vi "AnalogicMeas.vi"() -> ()   [LabVIEW 2017]
uses:
  DefDeType/ListeMachineEtats.ctl
  <vilib>/DAQmx/read.llb/DAQmx Read (Analog 1D Wfm NChan NSamp).vi
  DefDeType/WhichPath.ctl
  <vilib>/DAQmx/write.llb/DAQmx Write (Digital Bool 1Line 1Point).vi
  DefDeType/ClusterRefCtrlUSBB.ctl
  <vilib>/DAQmx/create/channels.llb/DAQmx Create Channel (DO-Digital Output).vi
  <vilib>/DAQmx/configure/trigger.llb/DAQmx Start Trigger (Digital Edge).vi
  <vilib>/DAQmx/configure/task.llb/DAQmx Configure Logging (TDMS).vi
panel:
  in  "Reprocess":bool
  in  "Calibration":bool
  out "Graph2":waveform(dbl)[](graph)
  in  "NextTest Num":u32
  out "num iteration":i32
  out "Acquisition Time":dbl(slide) max=10.0 scale=0.0..1000.0
  in  "ModifConfig":bool
  out "Test List":i32(listbox)=-1
  in  "Bouton Stop":bool
  in  "Bouton Rec":bool
  out "Projet :":string
  out "message":string
  in  "Bouton Quit":bool
  out "LoopTime":u32(graph)
  out "Graph1":waveform(dbl)[](graph)
  # "Analogic Measurements"
  # "Project"
  # "Actions"
  # "Test List"
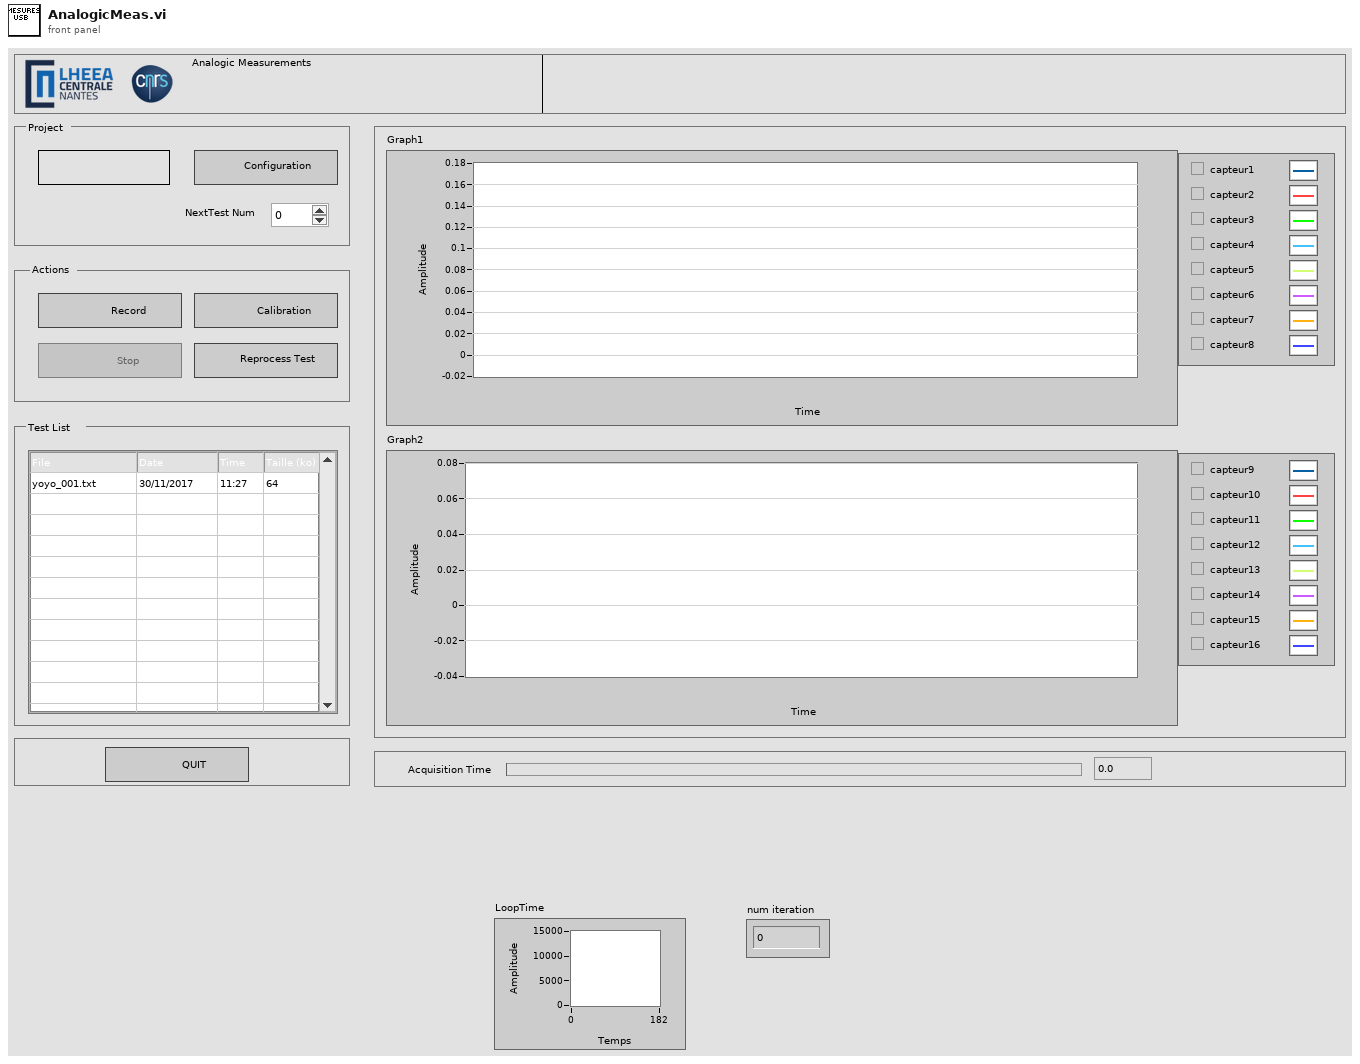
[diagram p1: front panel]
types:
  T1 = typedef "ClusterRefCtrlUSBB.ctl" = cluster{"Reprocess":refnum<vi>, "ModifConfig":refnum<vi>, "Bouton Rec":refnum<vi>, "Bouton Stop":refnum<vi>, "Bouton Quit":refnum<vi>, "Calibration":refnum<vi>, "Test List":refnum<vi>, "NextTest Num":refnum<vi>, "message":refnum<vi>}
  T2 = typedef "ListeMachineEtats.ctl" = enum16{"Init", "NewProj", "OpenProj", "InitLect", "Lect", "InitRec", "Rec", "Processing", "Quit"}
  T3 = cluster{"Graph2Index":i32[], "Graph1Index":i32[]}
  T4 = enum8{"Enabled", "Disabled", "Disabled and Grayed Out"}
  T5 = enum32{"Invalid", "Standard", "Closed", "Hidden", "Minimized", "Maximized"}
  T6 = typedef "WhichPath.ctl" = enum16{"DossierProjet", "Config", "Meas", "MeasPCI", "MeasCRIO1", "MeasCRIO2", "MeasQualisys", "MeasHBM", "MeasTDMS", "Fig", "Res"}
  T7 = typedef "WhichPath.ctl" = enum16{"DossierProjet", "Config", "Meas", "MeasSuitCase", "MeasOnBoard", "MeasQualisys", "MeasTDMS", "MeasHexapode", "MeasNortek", "Fig", "Res", "MeasUSB"}
  T8 = typedef "ConfigTotale.ctl" = cluster{"VoltageChannels":T9, "WheastoneBridgeChannels":T10, "Configuration":T11}
  T9 = typedef "VoltageChannels.ctl" = cluster{"ChannelNames":string[], "Sensitivity(Unit/V)":dbl[], "AutoZero":bool[], "ChannelUnits":string[], "Offsets(Units)":dbl[], "Graph Num":u8[]}
  T10 = typedef "WBridgeChannels.ctl" = cluster{"ChannelNames":string[], "Sensitivity(Unit/V)":dbl[], "AutoZero":bool[], "ChannelUnits":string[], "Offsets(Units)":dbl[], "Graph Num":u8[]}
  T11 = typedef "Configuration.ctl" = cluster{"AcqSamplingRate(Hz)":u32, "AcqTime(s)":u32, "Trigger":bool, "NbVoltageChannels":u32, "NbWBridgeChannels":u32, "Qualisys":bool, "Hexapode":bool, "FinalSamplingRate(Hz)":u32, "QualisysDataType":enum16{"6DOF", "3DTracking", "6DOF + 3D"}, "Nortek":bool, "HBM":bool}
  T12 = cluster{"Acquisition Time":refnum<vi>, "Graph1":refnum<vi>, "Graph2":refnum<vi>}
  T13 = typedef "MergeFileConfig.ctl" = cluster{"Test Num : ":u32, "Project :":string, "Qualisys file":path, "HBM file":path, "QualisysDataType":enum16{"6DOF", "3DTracking", "6DOF + 3D"}, "Qualisys":bool, "HBM":bool}
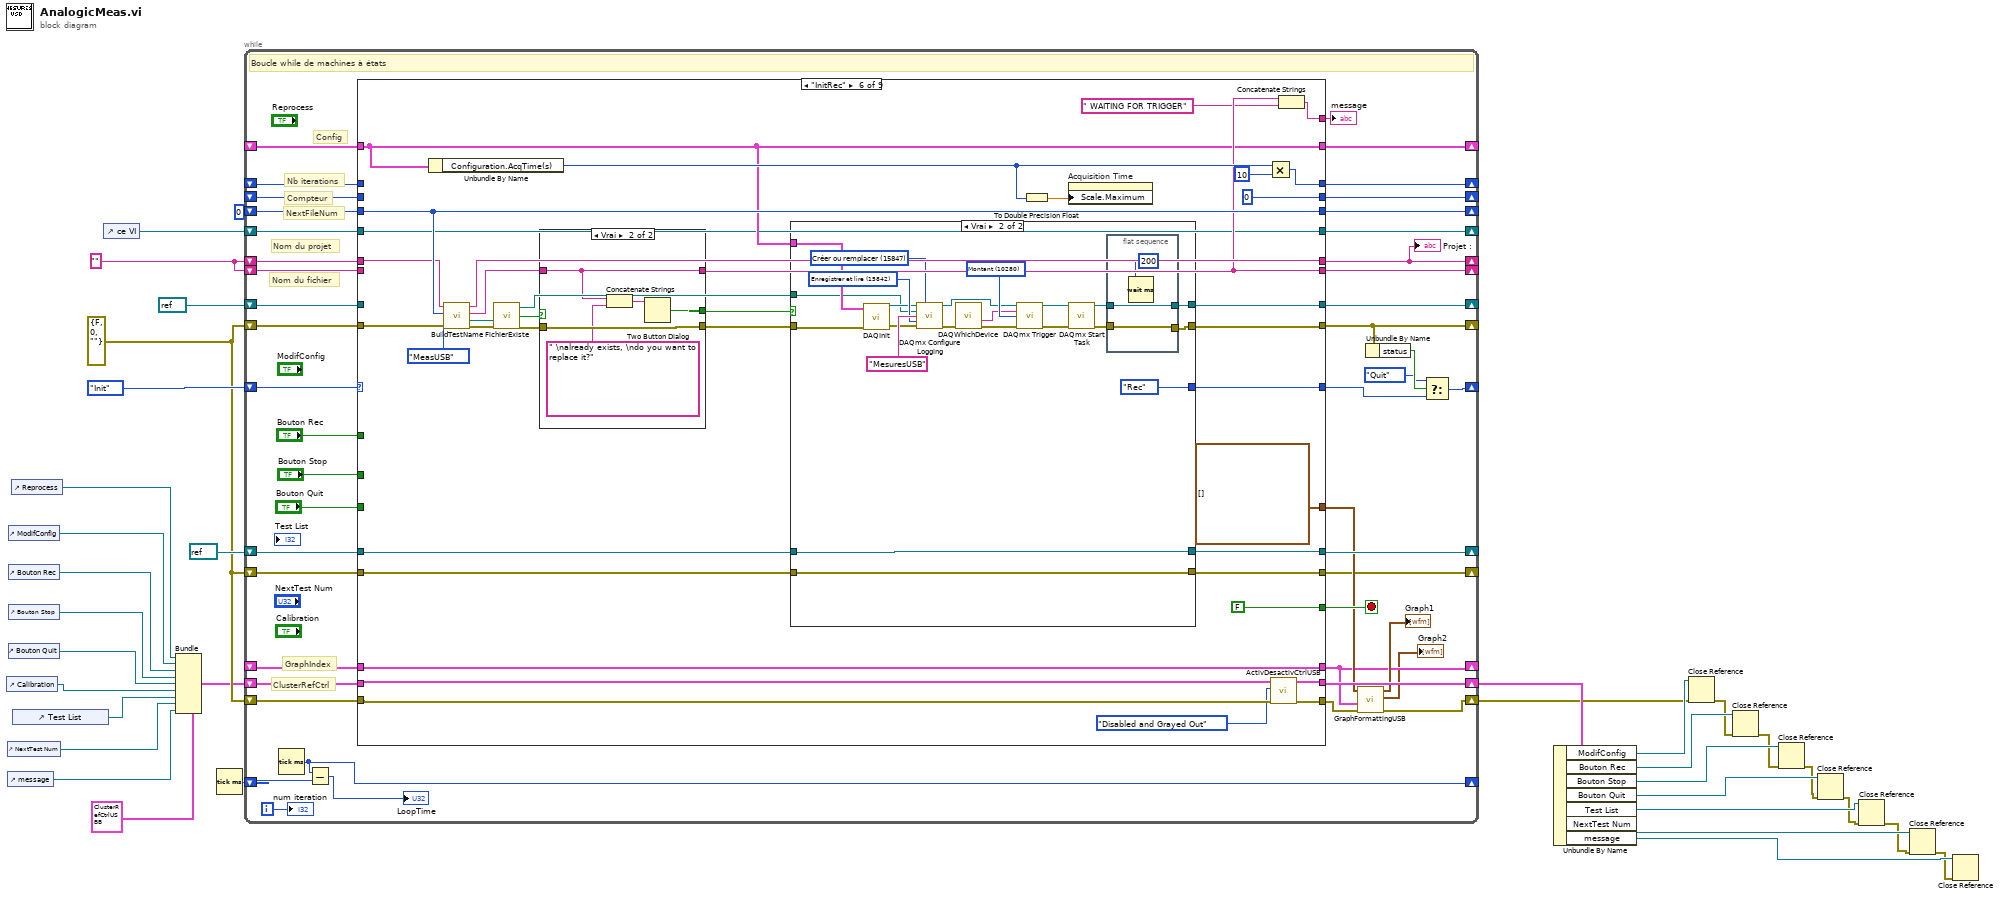
[diagram p0: block diagram]
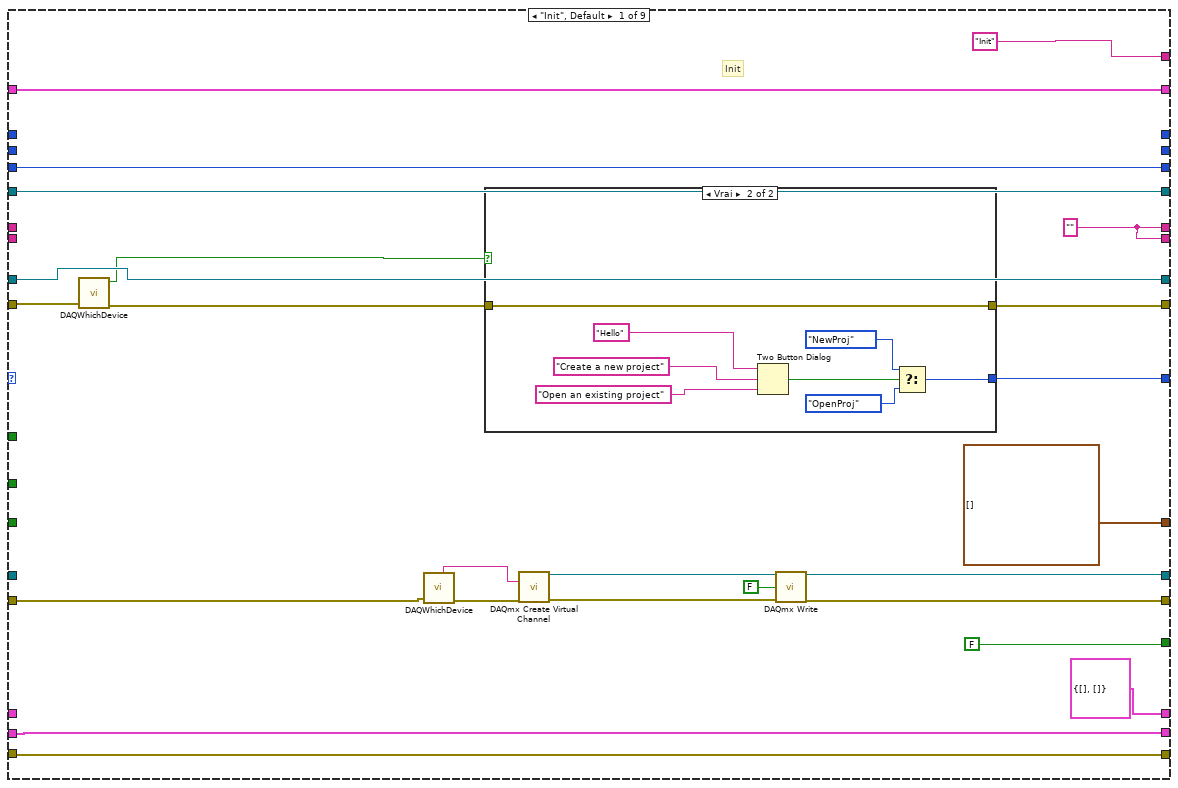
[diagram p2: hidden frame]
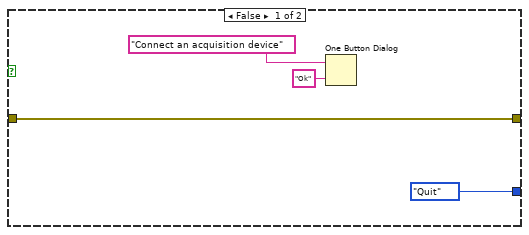
[diagram p3: hidden frame]
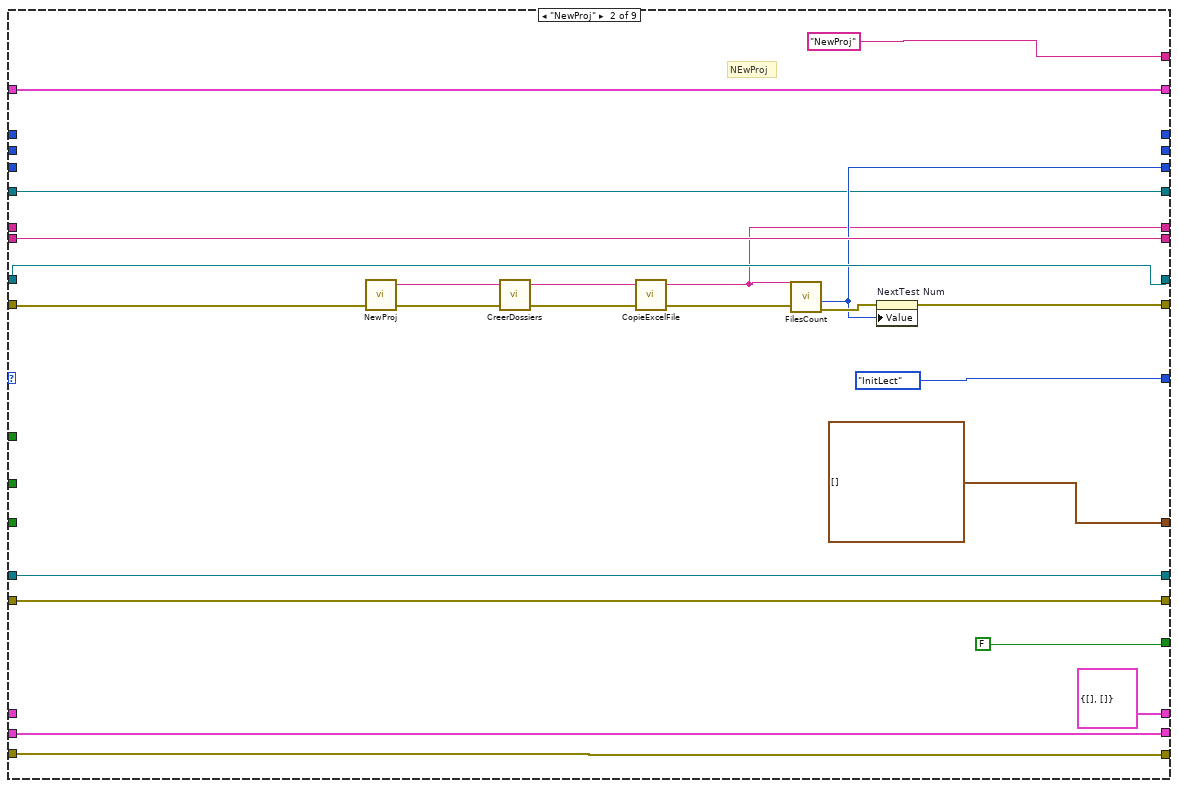
[diagram p4: hidden frame]
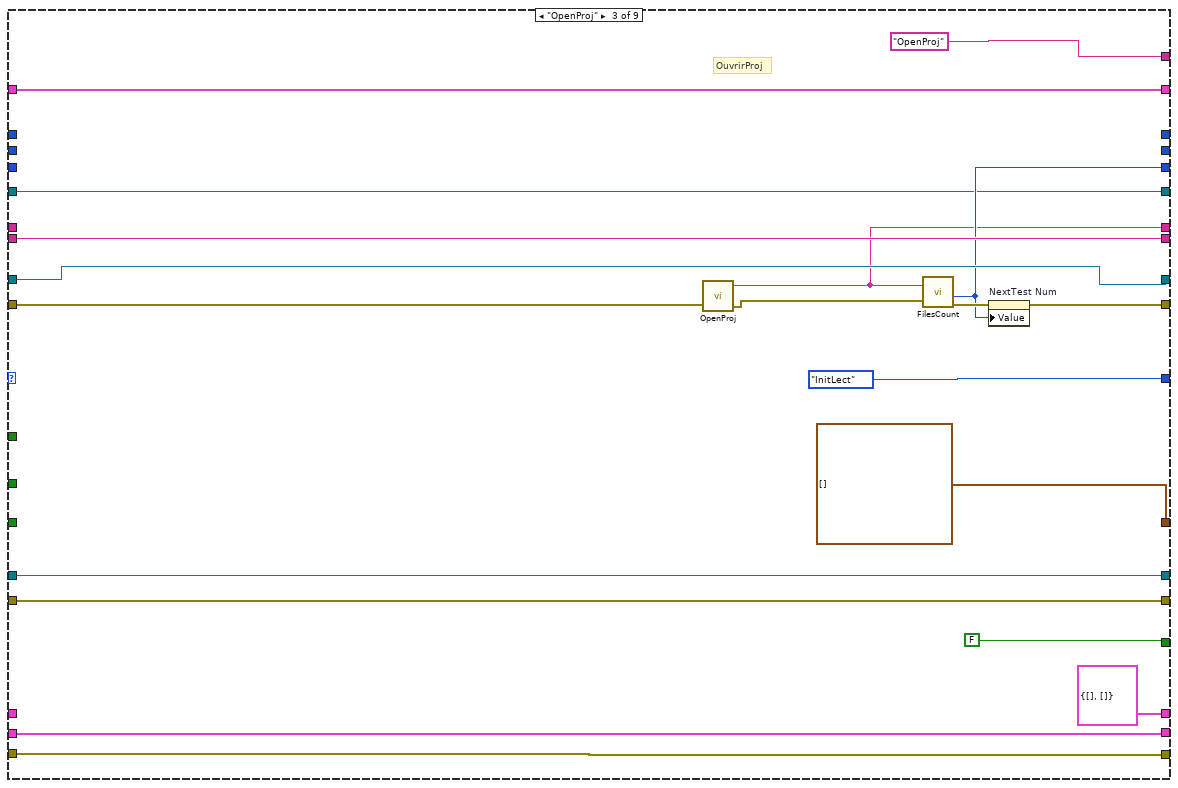
[diagram p5: hidden frame]
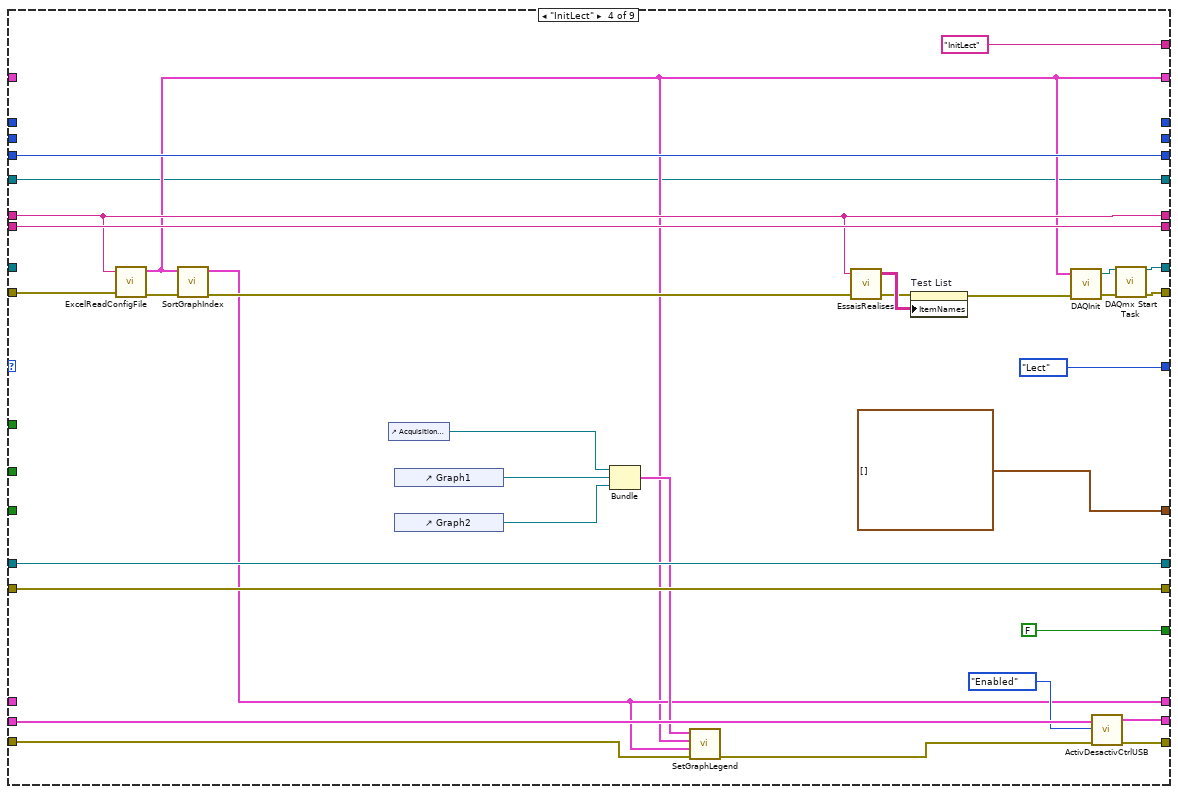
[diagram p6: hidden frame]
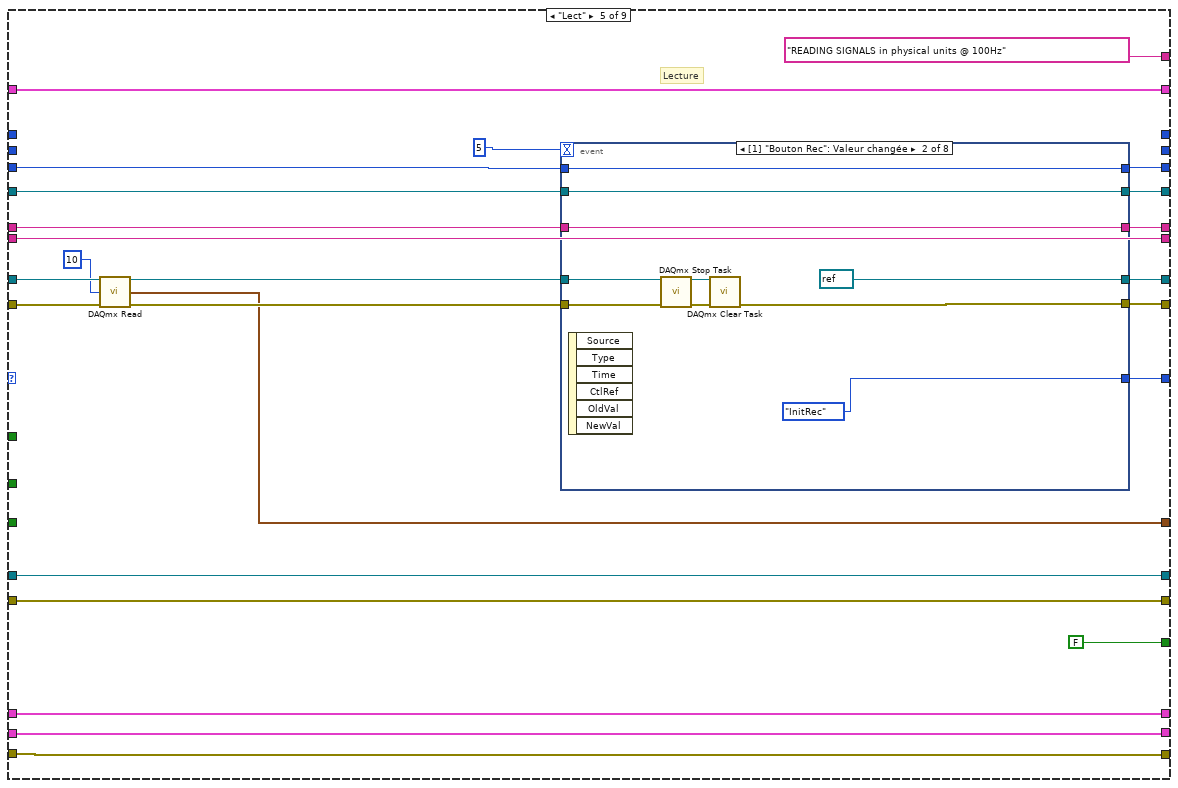
[diagram p7: hidden frame]
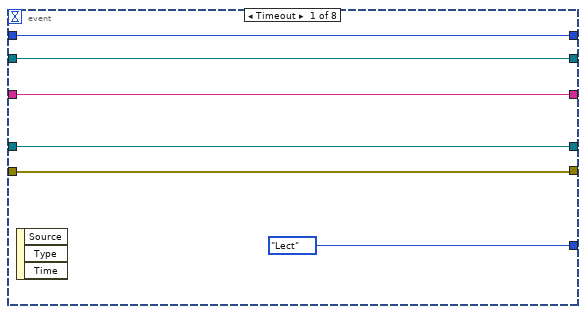
[diagram p8: hidden frame]
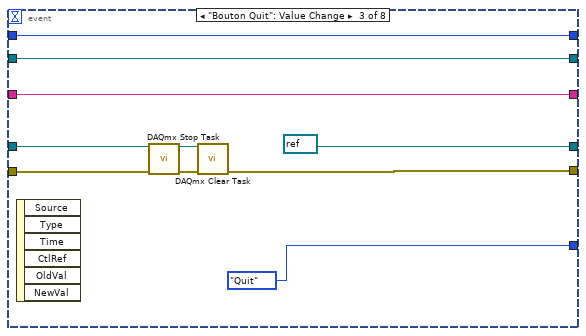
[diagram p9: hidden frame]
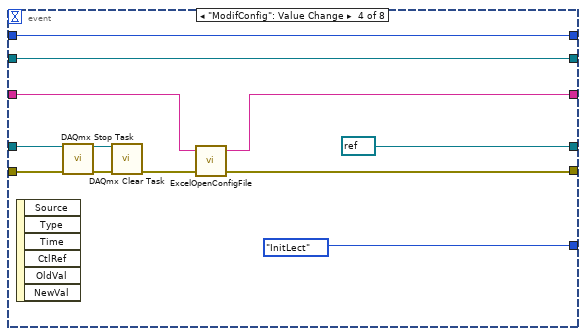
[diagram p10: hidden frame]
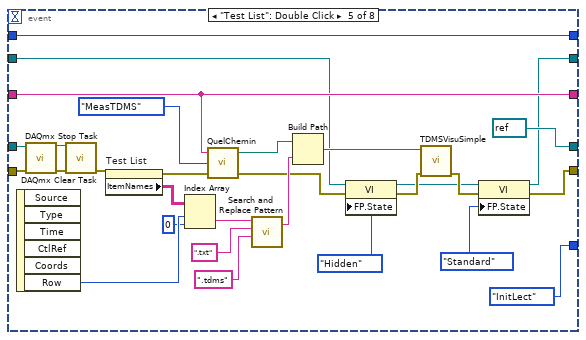
[diagram p11: hidden frame]
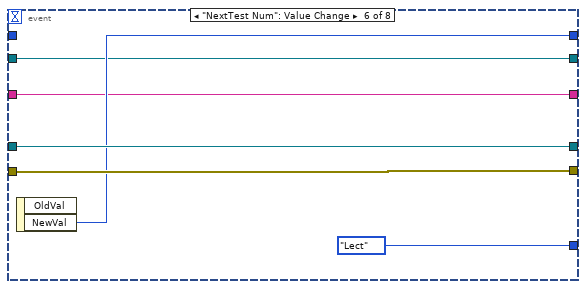
[diagram p12: hidden frame]
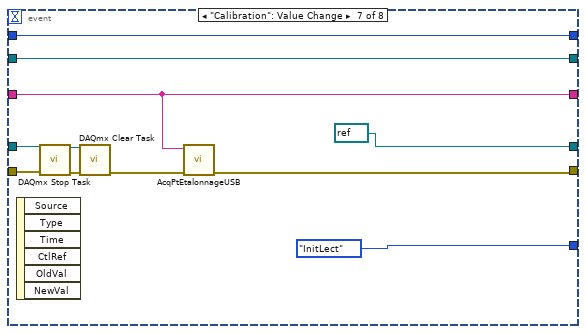
[diagram p13: hidden frame]
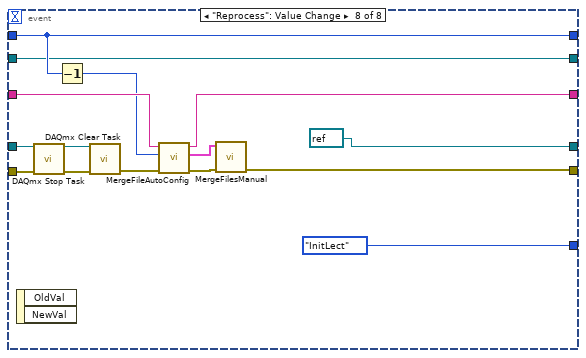
[diagram p14: hidden frame]
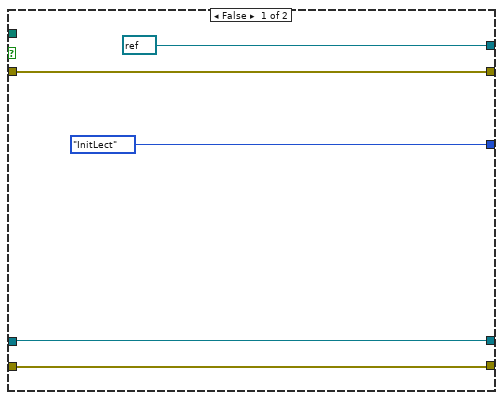
[diagram p15: hidden frame]
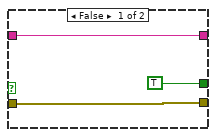
[diagram p16: hidden frame]
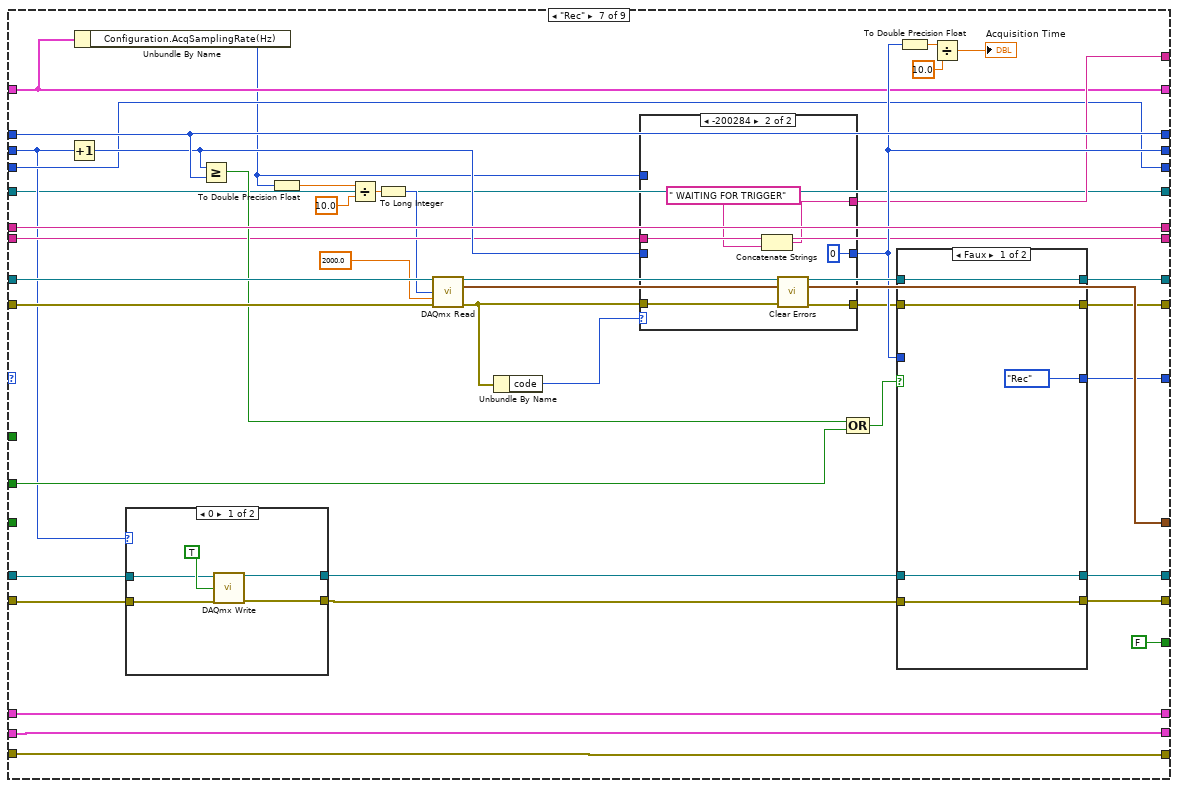
[diagram p17: hidden frame]
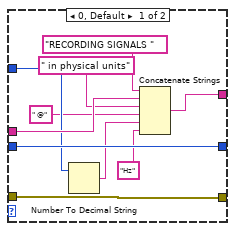
[diagram p19: hidden frame]
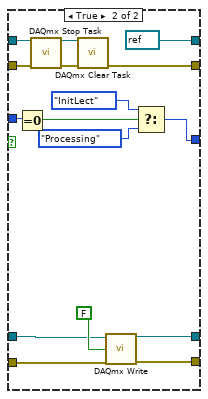
[diagram p20: hidden frame]
diagram:
  w29 = "" ("NomProjetOUT")
  w28 = errorcluster {"status"=FALSE, "code"=0, "source"=""} ("error out")
  n1 = control-ref of="Calibration"() -> (w5:refnum<vi>)
  n2 = control-ref of="NextTest Num"() -> (w22:refnum<vi>)
  n3 = control-ref of="message"() -> (w21:refnum<vi>)
  n4 = control-ref of="ModifConfig"() -> (w27:refnum<vi>)
  n5 = control-ref of="Bouton Rec"() -> (w26:refnum<vi>)
  n6 = control-ref of="Bouton Stop"() -> (w25:refnum<vi>)
  n7 = control-ref of="Bouton Quit"() -> (w24:refnum<vi>)
  n8 = control-ref of="Reprocess"() -> (w4:refnum<vi>)
  n9 = control-ref of="Test List"() -> (w23:refnum<vi>)
  n10 = control-ref of="ce VI"() -> (w1:refnum<vi>)
  n11 = Bundle(cluster=T1 {"Reprocess"=refnum, "ModifConfig"=refnum, "Bouton Rec"=refnum, "Bouton Stop"=refnum, "Bouton Quit"=refnum, "Calibration"=refnum, "Test List"=refnum, "NextTest Num"=refnum, "message"=refnum} ("ClusterRefCtrl"), "Reprocess"=w4, "ModifConfig"=w27, "Bouton Rec"=w26, "Bouton Stop"=w25, "Bouton Quit"=w24, "Calibration"=w5, "Test List"=w23, "NextTest Num"=w22, "message"=w21) -> (w2:T1)
  n12 = Tick Count (ms)() -> (millisecond timer value=w33:u32)
  n13 = while {
    shift-right: [w40] -> _
    shift-left: ListeMachineEtats."Init" ("ListeMachineEtats") -> [w61]
    shift-right: [w52] -> _
    shift-left: w29 -> [w79]
    shift-right: [w39] -> _
    shift-left: w28 -> [w78]
    shift-right: [w77] -> _
    shift-left: refnum<k21> refnum ("task out") -> [w76]
    shift-right: [w71] -> _
    shift-left: w29 -> [w70]
    shift-right: [w68] -> _
    shift-left: w33 -> [w69]
    shift-right: [w38] -> _
    shift-left: w28 -> [w66]
    shift-right: [w65] -> _
    shift-left: refnum<k21> refnum ("task out") -> [w64]
    shift-right: [w63] -> _
    shift-left: _ -> [w62]
    shift-right: [w37] -> w12
    shift-left: w28 -> [w60]
    shift-right: [w59] -> _
    shift-left: _ -> [w58]
    shift-right: [w57] -> _
    shift-left: _ -> [w56]
    shift-right: [w54] -> _
    shift-left: u32 0 ("NewVal") -> [w53]
    shift-right: [w50] -> w20
    shift-left: w2 -> [w51]
    shift-right: [w45] -> _
    shift-left: _ -> [w49]
    shift-right: [w35] -> _
    shift-left: w1 -> [w36]
    i -> [w55]
    stop <- w75 stop-if-true
    # "ClusterRefCtrl"
    # "GraphIndex"
    # "NextFileNum"
    # "Compteur"
    # "Nb iterations"
    # "Config"
    # "Nom du fichier"
    # "Nom du projet"
    # "Boucle while de machines à états"
    n14 = Tick Count (ms)() -> (millisecond timer value=w68:u32)
    n15 = Subtract(x=w68, y=w69) -> (x-y=→"LoopTime":u32)
    n16 = case shown="\"InitRec\"" w61 {
      tunnel: [w104 ListeMachineEtats."InitLect" ("ListeMachineEtats") ListeMachineEtats."InitLect" ("ListeMachineEtats") ListeMachineEtats."Lect" ("ListeMachineEtats") w205 w344 w425 ListeMachineEtats."InitLect" ("ListeMachineEtats") ListeMachineEtats."Init" ("ListeMachineEtats")] -> w42
      tunnel: ["Init" ("message") "NewProj" ("message") "OpenProj" ("message") "InitLect" ("message") "READING SIGNALS in physical units @ 100Hz" ("message") w343 w406 "Data Processing" ("message") "Quitter" ("message")] -> w80
      tunnel: [w93 w120 w143 w176 w198 w331 w424 w485 w528] -> w52
      tunnel: w79 -> [_ _ _ w176 w204 w332 w424 w489 _]
      tunnel: [w96 w123 w145 w183 w207 w349 w426 w494 w507] -> w39
      tunnel: w78 -> [w99 w134 w157 w177 w213 w335 w432 w490 w513]
      tunnel: [w102 w133 w156 w185 w206 w350 w427 refnum<k21> refnum ("task out") refnum<k21> refnum ("task out")] -> w77
      tunnel: w76 -> [w102 w133 w156 _ w214 _ w431 _ w512]
      tunnel: [waveform(dbl)[] [] ("data") waveform(dbl)[] [] ("data") waveform(dbl)[] [] ("data") waveform(dbl)[] [] ("data") w197 waveform(dbl)[] [] ("data") w430 waveform(dbl)[] [] ("data") waveform(dbl)[] [] ("data")] -> w47
      tunnel: [FALSE FALSE FALSE FALSE FALSE FALSE FALSE FALSE TRUE] -> w75
      tunnel: "Bouton Quit" -> [_ _ _ _ _ _ _ _ _]
      tunnel: "Bouton Rec" -> [_ _ _ _ _ _ _ _ _]
      tunnel: "Bouton Stop" -> [_ _ _ _ _ _ w423 _ _]
      tunnel: [w93 w130 w153 w182 w210 w329 w407 w501 w528] -> w71
      tunnel: w70 -> [_ w130 w153 w182 w210 _ w407 w501 _]
      tunnel: w66 -> [w90 w129 w152 w175 w196 w326 w399 w500 w519]
      tunnel: [w87 w128 w151 w174 w195 w323 w396 w487 refnum<k21> refnum ("task out")] -> w65
      tunnel: [w86 w129 w152 w175 w196 w324 w397 w500 w518] -> w38
      tunnel: w64 -> [_ w128 w151 w174 w195 w325 w400 w487 w520]
      tunnel: [w95 w127 w150 w161 w202 w327 w402 w497 w526] -> w63
      tunnel: w62 -> [w95 w127 w150 _ w202 w327 w402 w497 w526]
      tunnel: w60 -> [w94 w126 w149 w165 w203 w321 w421 w499 w525]
      tunnel: [w94 w126 w149 w173 w203 w322 w421 w499 w525] -> w48
      tunnel: [_ _ _ _ _ w346 w417 w491 w523] -> w59
      tunnel: w58 -> [_ _ _ _ _ _ w417 _ _]
      tunnel: [_ _ _ _ _ u32 0 ("y") w410 w491 w523] -> w57
      tunnel: w56 -> [_ _ _ _ _ _ w398 _ _]
      tunnel: [w82 w122 w144 w180 w201 w342 w405 w493 w523] -> w54
      tunnel: w53 -> [w82 _ _ w180 w200 w342 w405 w483 _]
      tunnel: w51 -> [w84 w119 w142 w172 w194 w318 w393 w479 w517]
      tunnel: [w84 w119 w142 w171 w194 w319 w393 w479 w517] -> w50
      tunnel: [T3 {"Graph2Index"=[], "Graph1Index"=[]} ("GraphIndex") T3 {"Graph2Index"=[], "Graph1Index"=[]} ("GraphIndex") T3 {"Graph2Index"=[], "Graph1Index"=[]} ("GraphIndex") w162 w193 w317 w392 w478 T3 {"Graph2Index"=[], "Graph1Index"=[]} ("GraphIndex")] -> w45
      tunnel: w49 -> [_ _ _ _ w193 w317 w392 w478 _]
      tunnel: w36 -> [w81 w117 w140 w159 w192 w315 w391 w477 w509]
      tunnel: [w81 w117 w140 w159 w191 w315 w391 w477 w506] -> w35
      frame "Init", Default {
        w93 = "" ("NomProjet")
        # "Init"
        n17 = call "DAQWhichDevice.vi"("error in"=w99) -> ("error out"=w97:errorcluster, "OK?"=w98:bool)  [unwired: 1 in, 5 out]
        n18 = call "DAQWhichDevice.vi"("error in"=w90) -> ("error out"=w92:errorcluster, "DigitalInputFinAcq"=w91:tag)  [unwired: 1 in, 5 out]
        n19 = case shown="Vrai" w98 {
          tunnel: [ListeMachineEtats."Quit" ("ListeMachineEtats") w112] -> w104
          tunnel: w97 -> [w108 w111]
          tunnel: [w108 w111] -> w96
          frame False {
            n20 = One Button Dialog(message="Connect an acquisition device", button name ("OK")="Ok" ("nom du bouton (\"OK\")")) -> ()  [unwired: 1 out]
          }
          frame True {
            n21 = Two Button Dialog(message="Hello", 1:"Open an existing project" ("Nom du bouton F (\"Annuler\")"), 2:"Create a new project" ("Nom du bouton V (\"OK\")")) -> (T button?=w113:bool)
            n22 = Select(t=ListeMachineEtats."NewProj" ("ListeMachineEtats"), s=w113, f=ListeMachineEtats."OpenProj" ("ListeMachineEtats")) -> (s? t:f=w112:T2)
          }
        }
        n23 = call-poly <vilib>:"DAQmx Create Virtual Channel.vi"("lines"=w91, "error in"=w92) -> ("task out"=w89:refnum<k21>, "error out"=w88:errorcluster)  [unwired: 12 in]
        n24 = call-poly <vilib>:"DAQmx Write.vi"("task/channels in"=w89, "data"=FALSE, "error in"=w88) -> ("task out"=w87:refnum<k21>, "error out"=w86:errorcluster)  [unwired: 10 in, 1 out]
      }
      frame "NewProj" {
        # "NEwProj"
        n25 = call "NewProj.vi"("entrée d'erreur"=w134) -> ("sortie d'erreur"=w137:errorcluster, "NomProjet"=w138:string)  [unwired: 3 in]
        n26 = call "CreerDossiers.vi"("Entrée d'erreur"=w137, "NomProjet"=w138) -> ("error out"=w136:errorcluster, "NomProjetOut"=w135:string)  [unwired: 2 in]
        n27 = call "CopieExcelFile.vi"("Entrée d'erreur"=w136, "NomProjet"=w135) -> ("sortie d'erreur"=w121:errorcluster, "NomProjetOut"=w120:string)  [unwired: 2 in]
        n28 = call "FilesCount.vi"("NomProjet"=w120, "entrée d'erreur"=w121) -> ("NextTestNum"=w122:u32, "sortie d'erreur"=w124:errorcluster)  [unwired: 4 out]
        n29 = property on="NextTest Num" class="NumNb (strict)"(error in=w124, "Value"=w122) -> (error out=w123:errorcluster)  [unwired: 1 in, 1 out]
      }
      frame "OpenProj" {
        # "OuvrirProj"
        n30 = call "OpenProj.vi"("entrée d'erreur"=w157) -> ("sortie d'erreur"=w147:errorcluster, "NomProjet"=w143:string)  [unwired: 3 in]
        n31 = call "FilesCount.vi"("NomProjet"=w143, "entrée d'erreur"=w147) -> ("NextTestNum"=w144:u32, "sortie d'erreur"=w146:errorcluster)  [unwired: 4 out]
        n32 = property on="NextTest Num" class="NumNb (strict)"(error in=w146, "Value"=w144) -> (error out=w145:errorcluster)  [unwired: 1 in, 1 out]
      }
      frame "InitLect" {
        n33 = call "ExcelReadConfigFile.vi"("NomProjet"=w176, "error in (no error)"=w177) -> ("ConfigurationTotale"=w161:T8, "error out"=w169:errorcluster)  [unwired: 3 in]
        n34 = call "SortGraphIndex.vi"("Error In"=w169, "ConfigurationTotale"=w161) -> ("Error Out"=w168:errorcluster, "GraphIndex"=w162:T3)  [unwired: 4 in]
        n35 = control-ref of="Acquisition Time"() -> (w167:refnum<vi>)
        n36 = control-ref of="Graph1"() -> (w166:refnum<vi>)
        n37 = control-ref of="Graph2"() -> (w160:refnum<vi>)
        n38 = Bundle("Acquisition Time"=w167, "Graph1"=w166, "Graph2"=w160) -> (w163:T12)  [unwired: 1 in]
        n39 = call "SetGraphLegend.vi"("error in (no error)"=w165, "GraphIndex"=w162, "ConfigTotale"=w161, "ClusterRefGraphs"=w163) -> ("error out"=w164:errorcluster)  [unwired: 3 in]
        n40 = call "EssaisRealises.vi"("entrée d'erreur (pas d'erreur)"=w168, "NomProjet"=w176) -> ("sortie d'erreur"=w178:errorcluster, "InfosFichiers"=w179:string[][])  [unwired: 2 in]
        n41 = property on="Test List" class="ListeMCol (strict)"(error in=w178, "ItemNames"=w179) -> (error out=w187:errorcluster)  [unwired: 1 in, 1 out]
        n42 = call "DAQInit.vi"("error in"=w187, "configInput"=w161) -> ("error out"=w184:errorcluster, "task out"=w186:refnum<k21>)  [unwired: 2 in]
        n43 = call "ActivDesactivCtrlUSB.vi"("error in (no error)"=w164, "Disabled"=T4."Enabled", "ClusterRefCtrl_IN"=w172) -> ("error out"=w173:errorcluster, "ClusterRefCtrl_OUT"=w171:T1)  [unwired: 3 in]
        n44 = call <vilib>:"DAQmx Start Task.vi"("task/channels in"=w186, "error in"=w184) -> ("task out"=w185:refnum<k21>, "error out"=w183:errorcluster)  [unwired: 12 in]
      }
      frame "Lect" {
        # "Lecture"
        n45 = call-poly <vilib>:"DAQmx Read.vi"("task/channels in"=w214, "number of samples per channel"=10, "error in"=w213) -> ("task out"=w209:refnum<k21>, "data"=w197:waveform(dbl)[], "error out"=w199:errorcluster)  [unwired: 10 in]
        n46 = event shown="[1] \"Bouton Rec\": Valeur changée" {
          selector: _ -> [_ _ _ _ _ _ _ _]
          dyn-events: _ -> [_ _ _ _ _ _ _ _]
          timeout: 5 -> [_ _ _ _ _ _ _ _]
          tunnel: w199 -> [w221 w229 w239 w250 w269 w287 w297 w309]
          tunnel: w209 -> [w220 w228 w238 w251 w272 w288 w298 w310]
          tunnel: [w221 w227 w237 w247 w257 w287 w291 w302] -> w207
          tunnel: [w220 refnum<k21> refnum ("task out") refnum<k21> refnum ("task out") refnum<k21> refnum ("task out") refnum<k21> refnum ("task out") w288 refnum<k21> refnum ("task out") refnum<k21> refnum ("task out")] -> w206
          tunnel: [ListeMachineEtats."Lect" ("ListeMachineEtats") ListeMachineEtats."InitRec" ("ListeMachineEtats") ListeMachineEtats."Quit" ("ListeMachineEtats") ListeMachineEtats."InitLect" ("ListeMachineEtats") ListeMachineEtats."InitLect" ("ListeMachineEtats") ListeMachineEtats."Lect" ("ListeMachineEtats") ListeMachineEtats."InitLect" ("ListeMachineEtats") ListeMachineEtats."InitLect" ("ListeMachineEtats")] -> w205
          tunnel: w204 -> [w217 w223 w233 w246 w266 w284 w292 w308]
          tunnel: [w218 w224 w234 w244 w267 w285 w290 w301] -> w201
          tunnel: w200 -> [w218 w224 w234 w244 w267 _ w290 w301]
          tunnel: [w217 w223 w233 w243 w266 w284 w292 w303] -> w198
          tunnel: w192 -> [w216 w222 w232 w242 w260 w283 w289 w300]
          tunnel: [w216 w222 w232 w242 w254 w283 w289 w300] -> w191
          event Timeout {
            n47 = event-data() -> ()  [unwired: 1 in, 3 out]
          }
          event "Bouton Rec": Value Change {
            n48 = event-data() -> ()  [unwired: 1 in, 6 out]
            n49 = call <vilib>:"DAQmx Stop Task.vi"("task/channels in"=w228, "error in"=w229) -> ("task out"=w230:refnum<k21>, "error out"=w231:errorcluster)  [unwired: 12 in]
            n50 = call <vilib>:"DAQmx Clear Task.vi"("task in"=w230, "error in"=w231) -> ("error out"=w227:errorcluster)  [unwired: 13 in]
          }
          event "Bouton Quit": Value Change {
            n51 = event-data() -> ()  [unwired: 1 in, 6 out]
            n52 = call <vilib>:"DAQmx Stop Task.vi"("task/channels in"=w238, "error in"=w239) -> ("task out"=w240:refnum<k21>, "error out"=w241:errorcluster)  [unwired: 12 in]
            n53 = call <vilib>:"DAQmx Clear Task.vi"("task in"=w240, "error in"=w241) -> ("error out"=w237:errorcluster)  [unwired: 13 in]
          }
          event "ModifConfig": Value Change {
            n54 = event-data() -> ()  [unwired: 1 in, 6 out]
            n55 = call <vilib>:"DAQmx Stop Task.vi"("task/channels in"=w251, "error in"=w250) -> ("task out"=w252:refnum<k21>, "error out"=w253:errorcluster)  [unwired: 12 in]
            n56 = call <vilib>:"DAQmx Clear Task.vi"("task in"=w252, "error in"=w253) -> ("error out"=w248:errorcluster)  [unwired: 13 in]
            n57 = call "ExcelOpenConfigFile.vi"("error in (no error)"=w248, "NomProjet"=w246) -> ("sortie d'erreur"=w247:errorcluster, "NomProjetOut"=w243:string)  [unwired: 2 in]
          }
          event "Test List": Double Click {
            n58 = event-data() -> ("Row"=w281:i32)  [unwired: 1 in, 5 out]
            n59 = call <vilib>:"DAQmx Stop Task.vi"("task/channels in"=w272, "error in"=w269) -> ("task out"=w271:refnum<k21>, "error out"=w270:errorcluster)  [unwired: 12 in]
            n60 = call <vilib>:"DAQmx Clear Task.vi"("task in"=w271, "error in"=w270) -> ("error out"=w273:errorcluster)  [unwired: 13 in]
            n61 = property on="Test List" class="ListeMCol (strict)"(error in=w273) -> (error out=w276:errorcluster, "ItemNames"=w282:string[][])  [unwired: 1 in, 1 out]
            n62 = Index Array(array=w282, index (row)=w281, index (col)=0 ("indice désactivé (col)")) -> (element=w277:string)
            n63 = call "QuelChemin.vi"("Entrée d'erreur"=w276, "WhichPath?"=WhichPath."MeasTDMS", "NomProjet"=w266) -> ("Sortie d'erreur"=w262:errorcluster, "SurDisqueLocal"=w275:path)  [unwired: 1 out]
            n64 = call <vilib>:"Search and Replace Pattern.vi"("string"=w277, "regular expression (\"\")"=".txt" ("regular expression (\"\")"), "replace string (\"\")"=".tdms" ("replace string (\"\")")) -> ("result string"=w263:string)  [unwired: 2 in, 1 out]
            n65 = Build Path(base path=w275, name or relative path=w263) -> (appended path=w264:path)
            n66 = property class="VI"(reference=w260, error in=w262, "FP.State"=T5."Hidden" ("Fenêtre face-avant:État")) -> (reference out=w255:refnum<vi>, error out=w261:errorcluster)
            n67 = call "TDMSVisuSimple.vi"("entrée d'erreur"=w261, "chemin du fichier"=w264) -> ("sortie d'erreur"=w258:errorcluster)  [unwired: 5 in]
            n68 = property class="VI"(reference=w255, error in=w258, "FP.State"=T5."Standard" ("Fenêtre face-avant:État")) -> (reference out=w254:refnum<vi>, error out=w257:errorcluster)
          }
          event "NextTest Num": Value Change {
            n69 = event-data() -> ("NewVal"=w285:u32)  [unwired: 1 in, 1 out]
          }
          event "Calibration": Value Change {
            n70 = event-data() -> ()  [unwired: 1 in, 6 out]
            n71 = call <vilib>:"DAQmx Stop Task.vi"("task/channels in"=w298, "error in"=w297) -> ("task out"=w299:refnum<k21>, "error out"=w296:errorcluster)  [unwired: 12 in]
            n72 = call <vilib>:"DAQmx Clear Task.vi"("task in"=w299, "error in"=w296) -> ("error out"=w295:errorcluster)  [unwired: 13 in]
            n73 = call "AcqPtEtalonnageUSB.vi"("entrée d'erreur"=w295, "Projet"=w292) -> ("sortie d'erreur"=w291:errorcluster)  [unwired: 5 in]
          }
          event "Reprocess": Value Change {
            n74 = event-data() -> ()  [unwired: 1 in, 2 out]
            n75 = call <vilib>:"DAQmx Stop Task.vi"("task/channels in"=w310, "error in"=w309) -> ("task out"=w312:refnum<k21>, "error out"=w311:errorcluster)  [unwired: 12 in]
            n76 = Decrement(x=w301) -> (x-1=w306:u32)
            n77 = call <vilib>:"DAQmx Clear Task.vi"("task in"=w312, "error in"=w311) -> ("error out"=w307:errorcluster)  [unwired: 13 in]
            n78 = call "MergeFileAutoConfig.vi"("error in (no error)"=w307, "test num"=w306, "ProjetIN"=w308) -> ("error out"=w305:errorcluster, "MergeFileConfigOUT"=w304:T13, "ProjetOUT"=w303:string)  [unwired: 2 in]
            n79 = call "MergeFilesManual.vi"("Error In"=w305, "MergeFileConfINPUT"=w304) -> ("sortie d'erreur"=w302:errorcluster)  [unwired: 5 in]
          }
        }
      }
      frame "InitRec" {
        n80 = Unbundle By Name(w327) -> ("Configuration.AcqTime(s)"=w334:u32)
        n81 = call "BuildTestName.vi"("entrée d'erreur"=w335, "WhichPath?"=WhichPath."MeasUSB", "NextTestNum"=w342, "NomProjet"=w332) -> ("sortie d'erreur"=w341:errorcluster, "cheminProchainFichier"=w340:path, "NomProchainFichier"=w330:string, "NomProjetOut"=w331:string)  [unwired: 1 in]
        n82 = call "FichierExiste.vi"("entrée d'erreur (pas d'erreur)"=w341, "cheminProchainFichierRAW"=w340) -> ("sortie d'erreur"=w338:errorcluster, "Booléen"=w337:bool, "path out"=w336:path)  [unwired: 1 in]
        n83 = case shown="Vrai" w337 {
          tunnel: [w385 w390] -> w339
          tunnel: w338 -> [w385 w390]
          tunnel: [TRUE ("T button?") w387] -> w328
          tunnel: w330 -> [w383 w386]
          tunnel: [w383 w386] -> w329
          frame False {
          }
          frame True {
            n84 = Concatenate Strings(w386, " \nalready exists, \ndo you want to replace it?" ("chaîne")) -> (w388:string)
            n85 = Two Button Dialog(message=w388) -> (T button?=w387:bool)  [unwired: 2 in]
          }
        }
        n86 = case shown="Vrai" w328 {
          tunnel: [refnum<k21> refnum ("task out") w358] -> w350
          tunnel: [w356 w360] -> w349
          tunnel: [ListeMachineEtats."InitLect" ("ListeMachineEtats") ListeMachineEtats."Rec" ("ListeMachineEtats")] -> w344
          tunnel: w339 -> [w356 w362]
          tunnel: w336 -> [_ w363]
          tunnel: w327 -> [_ w364]
          tunnel: w326 -> [w354 w378]
          tunnel: [w354 w378] -> w324
          tunnel: [w353 w377] -> w323
          tunnel: w325 -> [w353 w377]
          frame False {
          }
          frame True {
            w376 = 10280 items=["Montant"=10280, "Descendant"=10171] ("edge")
            w368 = 15847 items=["Ouvrir"=10437, "Ouvrir ou créer"=15846, "Créer ou remplacer"=15847, "Créer"=15848] ("operation")
            w367 = 15842 items=["Off"=10231, "Enregistrer"=15844, "Enregistrer et lire"=15842] ("logging mode")
            n87 = call "DAQInit.vi"("error in"=w362, "configInput"=w364) -> ("error out"=w365:errorcluster, "task out"=w366:refnum<k21>)  [unwired: 2 in]
            n88 = call-poly <vilib>:"DAQmx Configure Logging.vi"("task/channels in"=w366, "operation"=w368, "file path"=w363, "group name"="MesuresUSB", "logging mode"=w367, "error in"=w365) -> ("task out"=w370:refnum<k21>, "error out"=w369:errorcluster)  [unwired: 8 in]
            n89 = call "DAQWhichDevice.vi"("error in"=w369) -> ("error out"=w374:errorcluster, "sourceTrig"=w375:tag)  [unwired: 1 in, 5 out]
            n90 = call-poly <vilib>:"DAQmx Trigger.vi"("task/channels in"=w370, "source"=w375, "edge"=w376, "error in"=w374) -> ("task out"=w372:refnum<k21>, "error out"=w371:errorcluster)  [unwired: 10 in]
            n91 = call <vilib>:"DAQmx Start Task.vi"("task/channels in"=w372, "error in"=w371) -> ("task out"=w359:refnum<k21>, "error out"=w361:errorcluster)  [unwired: 12 in]
            n92 = flat-sequence {
              tunnel: [w382] -> w360
              tunnel: w361 -> [w382]
              tunnel: [w381] -> w358
              tunnel: w359 -> [w381]
              frame #0 {
                n93 = Wait (ms)(milliseconds to wait=u32 200 ("attente (ms)")) -> ()  [unwired: 1 out]
              }
            }
          }
        }
        n94 = To Double Precision Float(number=w334) -> (double precision float=w348:dbl)
        n95 = property on="Acquisition Time" class="Gliss (strict)"("Scale.Maximum"=w348) -> ()  [unwired: 2 in, 2 out]
        n96 = Multiply(x=w334, y=u32 10) -> (x*y=w346:u32)
        n97 = call "ActivDesactivCtrlUSB.vi"("error in (no error)"=w321, "Disabled"=T4."Disabled and Grayed Out", "ClusterRefCtrl_IN"=w318) -> ("error out"=w322:errorcluster, "ClusterRefCtrl_OUT"=w319:T1)  [unwired: 3 in]
        n98 = Concatenate Strings(w329, " WAITING FOR TRIGGER" ("message")) -> (w343:string)
      }
      frame "Rec" {
        n99 = Increment(x=w398) -> (x+1=w411:u32)
        n100 = Unbundle By Name(w402) -> ("Configuration.AcqSamplingRate(Hz)"=w401:u32)
        n101 = case shown="0" w398 {
          tunnel: w400 -> [w436 w439]
          tunnel: w399 -> [w435 w438]
          tunnel: [w434 w439] -> w394
          tunnel: [w433 w438] -> w395
          frame 0 {
            n102 = call-poly <vilib>:"DAQmx Write.vi"("task/channels in"=w436, "data"=TRUE, "error in"=w435) -> ("task out"=w434:refnum<k21>, "error out"=w433:errorcluster)  [unwired: 10 in, 1 out]
          }
          frame 1, Default {
          }
        }
        n103 = Greater Or Equal?(x=w411, y=w417) -> (x >= y?=w418:bool)
        n104 = To Double Precision Float(number=w401) -> (double precision float=w419:dbl)
        n105 = Divide(x=w419, y=10.0) -> (x/y=w404:dbl)
        n106 = To Long Integer(number=w404) -> (32bit integer=w403:i32)
        n107 = call-poly <vilib>:"DAQmx Read.vi"("task/channels in"=w431, "number of samples per channel"=w403, "timeout"=2000.0, "error in"=w432) -> ("task out"=w428:refnum<k21>, "data"=w430:waveform(dbl)[], "error out"=w409:errorcluster)  [unwired: 9 in]
        n108 = Unbundle By Name(w409) -> ("code"=w412:i32)
        n109 = case shown="-200284" w412 {
          tunnel: w411 -> [w449 _]
          tunnel: [w449 u32 0] -> w410
          tunnel: w409 -> [w448 w454]
          tunnel: [w448 w453] -> w408
          tunnel: w407 -> [w446 w452]
          tunnel: [w445 w451] -> w406
          tunnel: w401 -> [w443 _]
          frame 0, Default {
            n110 = Number To Decimal String(number=w443) -> (decimal integer string=w441:string)  [unwired: 1 in]
            n111 = Concatenate Strings("RECORDING SIGNALS " ("message"), w446, " in physical units" ("message"), " @" ("chaîne"), w441, "Hz" ("chaîne")) -> (w445:string)
          }
          frame -200284 {
            n112 = Concatenate Strings(w452, " WAITING FOR TRIGGER" ("message")) -> (w451:string)
            n113 = call <vilib>:"Clear Errors.vi"("error in (no error)"=w454) -> ("error out"=w453:errorcluster)  [unwired: 5 in, 1 out]
          }
        }
        n114 = Compound Arithmetic op=OR ("Opérateur arithmétique")(w418, w423) -> (w422:bool)
        n115 = case shown="Faux" w422 {
          tunnel: w428 -> [w460 w476]
          tunnel: [w460 refnum<k21> refnum ("task out")] -> w427
          tunnel: [w458 w472] -> w426
          tunnel: [ListeMachineEtats."Rec" ("ListeMachineEtats") w467] -> w425
          tunnel: w410 -> [_ w471]
          tunnel: w408 -> [w458 w466]
          tunnel: [w456 w464] -> w397
          tunnel: [w457 w463] -> w396
          tunnel: w395 -> [w456 w462]
          tunnel: w394 -> [w457 w461]
          frame False {
          }
          frame True {
            n116 = Equal To 0?(x=w471) -> (x = 0?=w470:bool)
            n117 = call <vilib>:"DAQmx Stop Task.vi"("task/channels in"=w476, "error in"=w466) -> ("task out"=w475:refnum<k21>, "error out"=w474:errorcluster)  [unwired: 12 in]
            n118 = call <vilib>:"DAQmx Clear Task.vi"("task in"=w475, "error in"=w474) -> ("error out"=w472:errorcluster)  [unwired: 13 in]
            n119 = call-poly <vilib>:"DAQmx Write.vi"("task/channels in"=w461, "data"=FALSE, "error in"=w462) -> ("task out"=w463:refnum<k21>, "error out"=w464:errorcluster)  [unwired: 10 in, 1 out]
            n120 = Select(t=ListeMachineEtats."InitLect" ("ListeMachineEtats"), s=w470, f=ListeMachineEtats."Processing" ("ListeMachineEtats")) -> (s? t:f=w467:T2)
          }
        }
        n121 = To Double Precision Float(number=w410) -> (double precision float=w416:dbl)
        n122 = Divide(x=w416, y=10.0) -> (x/y=→"Acquisition Time":dbl)
      }
      frame "Processing" {
        w491 = u32 0
        n123 = call "GetFilesUSB.vi"("error in (no error)"=w490, "Test Num :"=w483, "Project :"=w489) -> ("error out"=w486:errorcluster, "NomProjetOut"=w484:string)  [unwired: 3 in]
        n124 = call "MergeFileAutoConfig.vi"("error in (no error)"=w486, "test num"=w483, "ProjetIN"=w484) -> ("error out"=w482:errorcluster, "MergeFileConfigOUT"=w481:T13, "ProjetOUT"=w485:string)  [unwired: 2 in]
        n125 = call "MergeFilesManual.vi"("Error In"=w482, "MergeFileConfINPUT"=w481) -> ("sortie d'erreur"=w480:errorcluster)  [unwired: 5 in]
        n126 = call "EssaisRealises.vi"("entrée d'erreur (pas d'erreur)"=w480, "WhichPath?"=WhichPath."MeasTDMS", "NomProjet"=w485) -> ("sortie d'erreur"=w496:errorcluster, "InfosFichiers"=w492:string[][])  [unwired: 1 in]
        n127 = property on="Test List" class="ListeMCol (strict)"(error in=w496, "ItemNames"=w492) -> (error out=w495:errorcluster)  [unwired: 1 in, 1 out]
        n128 = Increment(x=w483) -> (x+1=w493:u32)
        n129 = property on="NextTest Num" class="NumNb (strict)"(error in=w495, "Value"=w493) -> (error out=w494:errorcluster)  [unwired: 1 in, 1 out]
      }
      frame "Quit" {
        w523 = u32 0
        w528 = "" ("NomProjet")
        n130 = call <vilib>:"DAQmx Stop Task.vi"("task/channels in"=w512, "error in"=w513) -> ("task out"=w515:refnum<k21>, "error out"=w514:errorcluster)  [unwired: 12 in]
        n131 = call <vilib>:"DAQmx Stop Task.vi"("task/channels in"=w520, "error in"=w519) -> ("task out"=w521:refnum<k21>, "error out"=w522:errorcluster)  [unwired: 12 in]
        n132 = call <vilib>:"DAQmx Clear Task.vi"("task in"=w515, "error in"=w514) -> ("error out"=w510:errorcluster)  [unwired: 13 in]
        n133 = call <vilib>:"DAQmx Clear Task.vi"("task in"=w521, "error in"=w522) -> ("error out"=w518:errorcluster)  [unwired: 13 in]
        n134 = call <vilib>:"Clear Errors.vi"("error in (no error)"=w510) -> ("error out"=w511:errorcluster)  [unwired: 5 in, 1 out]
        n135 = disable-structure shown="Activé" {
          disable-tunnel: w511 -> [w536 _]
          disable-tunnel: [w535 _] -> w508
          disable-tunnel: w509 -> [w534 _]
          disable-tunnel: [w533 _] -> w506
          frame Enabled {
            n136 = invoke class="VI" method="FA.Fermer"(reference=w534, error in=w536) -> (reference out=w533:refnum<vi>, error out=w535:errorcluster)  [unwired: 1 in, 1 out]
          }
          frame Disabled {
          }
        }
        n137 = Close Reference(reference=w506, error in (no error)=w508) -> (error out=w507:errorcluster)
      }
    }
    "message" <- w80
    "Projet :" <- w52
    n138 = call "GraphFormattingUSB.vi"("Error In"=w48, "GraphIndex"=w45, "dataIN"=w47) -> ("Error Out"=w37:errorcluster, "Graph2Data"=→"Graph2":waveform(dbl)[], "Graph1Data"=→"Graph1":waveform(dbl)[])  [unwired: 2 in]
    n139 = Unbundle By Name(w39) -> ("status"=w43:bool)
    n140 = Select(t=ListeMachineEtats."Quit" ("ListeMachineEtats"), s=w43, f=w42) -> (s? t:f=w40:T2)
    "num iteration" <- w55
  }
  n141 = Unbundle By Name(w20) -> ("ModifConfig"=w19:refnum<vi>, "Bouton Rec"=w18:refnum<vi>, "Bouton Stop"=w17:refnum<vi>, "Bouton Quit"=w16:refnum<vi>, "Test List"=w15:refnum<vi>, "NextTest Num"=w14:refnum<vi>, "message"=w13:refnum<vi>)
  n142 = Close Reference(reference=w19, error in (no error)=w12) -> (error out=w11:errorcluster)
  n143 = Close Reference(reference=w18, error in (no error)=w11) -> (error out=w10:errorcluster)
  n144 = Close Reference(reference=w17, error in (no error)=w10) -> (error out=w9:errorcluster)
  n145 = Close Reference(reference=w16, error in (no error)=w9) -> (error out=w8:errorcluster)
  n146 = Close Reference(reference=w15, error in (no error)=w8) -> (error out=w7:errorcluster)
  n147 = Close Reference(reference=w14, error in (no error)=w7) -> (error out=w6:errorcluster)
  n148 = Close Reference(reference=w13, error in (no error)=w6) -> ()  [unwired: 1 out]
